vi "start_camera_new.vi"(8 "error in (no error)":errorcluster, 10 "image type":T2, 11 "Camera settings":T1={"Gain"=1.0, "Exposure (s)"=0.05, "Preview binning"=2, "Capture binning"=0, "auto expose button"=FALSE} {"Capture binning" items=["1x1", "2x2", "4x4", "8x8"]; "Preview binning" items=["1x1", "2x2", "4x4", "8x8"]; "Exposure (s)" scale=1e-05..1000.0 scale format="%^#_1e"; "Gain" scale=0.451..21.5 scale format="%#_3g"}) -> (0 "error out":errorcluster, 2 "cameraId out":u32, 3 "Refnum out":T3)   [LabVIEW 2011]
uses:
  <vilib>/vision/Image Controls.llb/IMAQ Image.ctl
  typedefs/image_type.ctl
  typedefs/camera_settings_new.ctl
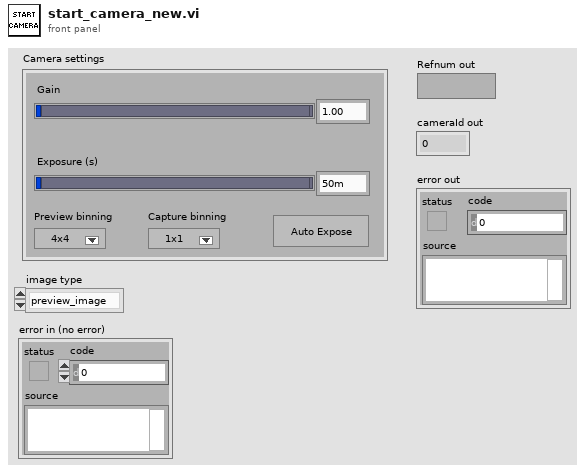
[diagram p1: front panel]
types:
  T1 = typedef "camera_settings_new.ctl" = cluster{"Gain":dbl, "Exposure (s)":dbl, "Preview binning":u16, "Capture binning":u16, "auto expose button":bool}
  T2 = typedef "image_type.ctl" = enum16{"preview_image", "capture_image"}
  T3 = typedef "IMAQ Image.ctl" = refnum<image>
  T4 = enum32{"gain", "offset", "exposure", "binning", "horizontal binning", "vertical binning", "readout speed", "trigger type", "lcd filter", "cooler", "exposure red", "exposure blue", "image format", "roi x", "roi y", "roi width", "roi height", "reserved1", "shutter state", "reserved2", "sync-b out", "reserved3", "intensifier gain", "trigger delay", "camera mode", "normalized gain", "normalized intenifier gain DB", "doPostProcessing", "postProcessGainRed", "postProcessGainGreen", "postProcessGainBlue", "postProcessBayerAlgorithm", "postProcessImageFormat", "fan", "blackout mode", "high sensitivity", "Readout Port", "EM Gain", "open delay", "close delay", "clearing mode"}
  T5 = typedef "Image Type" = u32
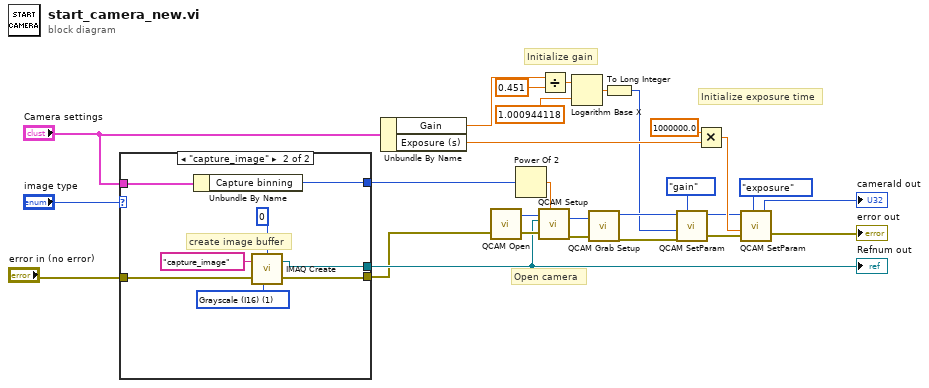
[diagram p0: block diagram]
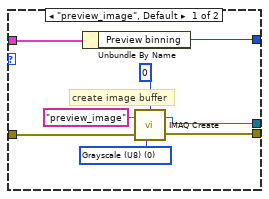
[diagram p2: hidden frame]
diagram:
  # "Initialize gain"
  # "Open camera"
  # "Initialize exposure time"
  n1 = case shown="\"capture_image\"" "image type" {
    tunnel: [w36 w43] -> w5
    tunnel: "Camera settings" -> [w35 w44]
    tunnel: [w31 w39] -> w3
    tunnel: "error in (no error)" -> [w30 w38]
    tunnel: [w29 w37] -> w1
    frame "preview_image", Default {
      w32 = T5 0 items=["Grayscale (U8)", "Grayscale (I16)", "Grayscale (SGL)", "Complex (CSG)", "RGB (U32)", "HSL (U32)", "RGB (U64)"] ("Image Type")
      # "create image buffer"
      n2 = Unbundle By Name(w35) -> ("Preview binning"=w36:u16)
      n3 = call "IMAQ Create"("Border Size"=0, "Image Name"="preview_image", "Image Type"=w32, "error in (no error)"=w30) -> ("New Image"=w31:T3, "error out"=w29:errorcluster)  [unwired: 1 in]
    }
    frame "capture_image" {
      w40 = T5 1 items=["Grayscale (U8)", "Grayscale (I16)", "Grayscale (SGL)", "Complex (CSG)", "RGB (U32)", "HSL (U32)", "RGB (U64)"] ("Image Type")
      # "create image buffer"
      n4 = Unbundle By Name(w44) -> ("Capture binning"=w43:u16)
      n5 = call "IMAQ Create"("Border Size"=0, "Image Name"="capture_image", "Image Type"=w40, "error in (no error)"=w38) -> ("New Image"=w39:T3, "error out"=w37:errorcluster)  [unwired: 1 in]
    }
  }
  "Refnum out" <- w3
  n6 = Unbundle By Name("Camera settings") -> ("Gain"=w10:dbl, "Exposure (s)"=w15:dbl)
  n7 = call <userlib>:"QCAM Open.vi"("error in (no error)"=w1) -> ("error out"=w22:errorcluster, "cameraId out"=w23:u32)  [unwired: 1 in]
  n8 = Power Of 2(x=w5) -> (2^x=w28:dbl)
  n9 = call <userlib>:"QCAM Setup.vi"("Optional Binning"=w28, "error in (no error)"=w22, "Image"=w3, "cameraId"=w23) -> ("error out"=w20:errorcluster, "cameraId out"=w21:u32)  [unwired: 3 in, 3 out]
  n10 = Divide(x=w10, y=0.451) -> (x/y=w11:dbl)
  n11 = Logarithm Base X(1:1.000944118 ("x"), 2:w11) -> (0:w8:dbl)
  n12 = call <userlib>:"QCAM Grab Setup.vi"("error in (no error)"=w20, "cameraId"=w21) -> ("error out"=w25:errorcluster, "cameraId out"=w24:u32)
  n13 = To Long Integer(number=w8) -> (32bit integer=w7:i32)
  n14 = call <userlib>:"QCAM SetParam.vi"("error in (no error)"=w25, "value"=w7, "parameter key"=T4."gain", "cameraId"=w24) -> ("error out"=w13:errorcluster, "cameraId out"=w14:u32)
  n15 = Multiply(x=1000000.0, y=w15) -> (x*y=w16:dbl)
  n16 = call <userlib>:"QCAM SetParam.vi"("error in (no error)"=w13, "value"=w16, "parameter key"=T4."exposure", "cameraId"=w14) -> ("error out"=→"error out":errorcluster, "cameraId out"=→"cameraId out":u32)
